vi "print.vi"(8 "error in (no error)":errorcluster, 10 "input":string, 11 "XMLPrettyPrinting in":refnum<class "XMLPrettyPrinting.lvclass">) -> (0 "error out":errorcluster, 2 "output":string, 3 "XMLPrettyPrinting out":refnum<class "XMLPrettyPrinting.lvclass">)   [LabVIEW 2011, in "Views.lvlib" / "ViewerTools.lvlib" / "XMLPrettyPrinting.lvclass"]
uses:
  XMLPrettyPrinting.lvclass
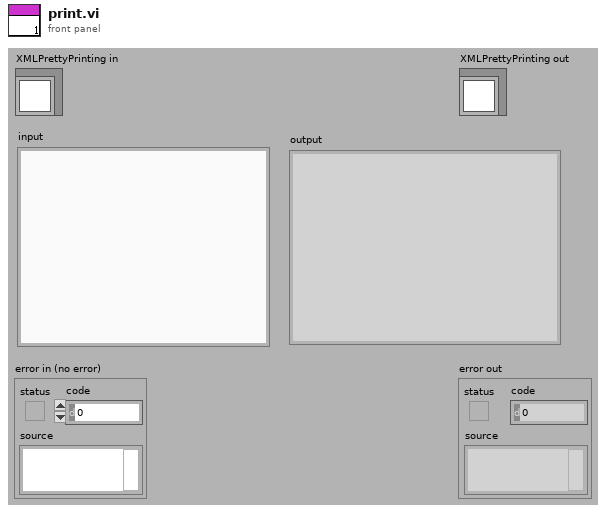
[diagram p1: front panel]
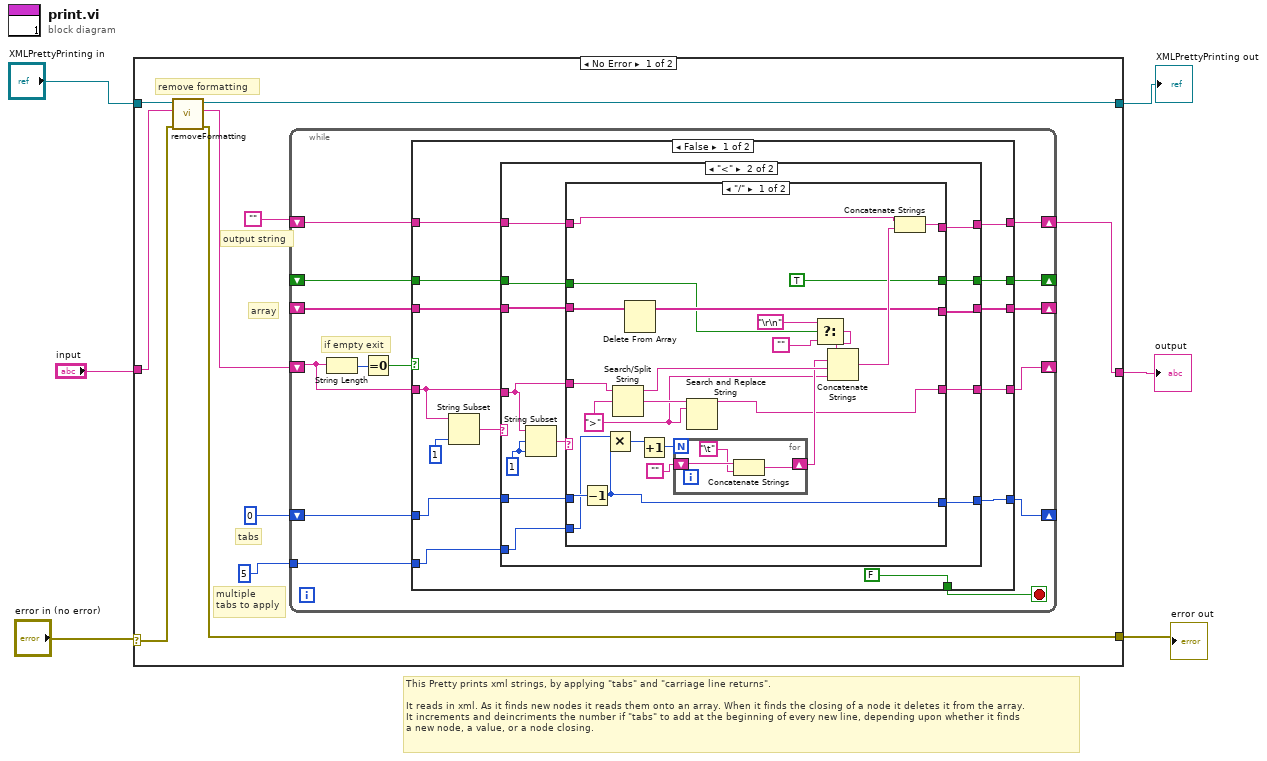
[diagram p0: block diagram]
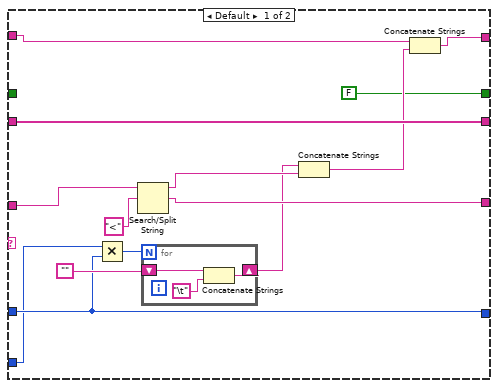
[diagram p2: hidden frame]
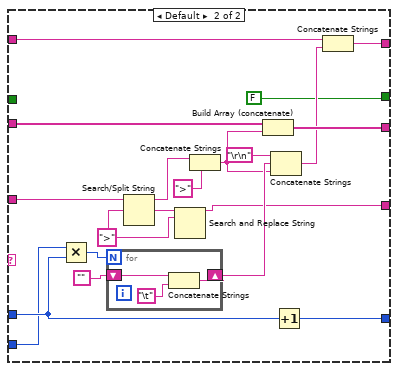
[diagram p3: hidden frame]
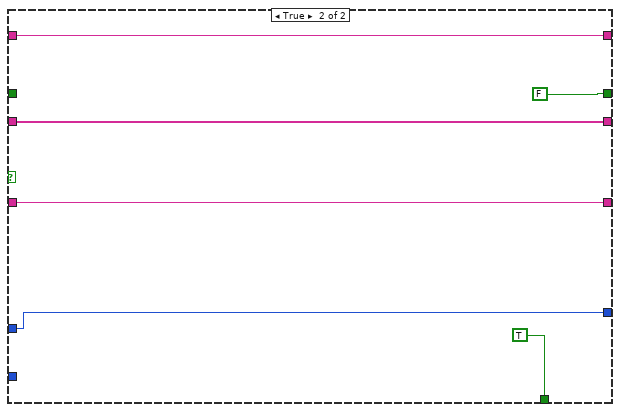
[diagram p4: hidden frame]
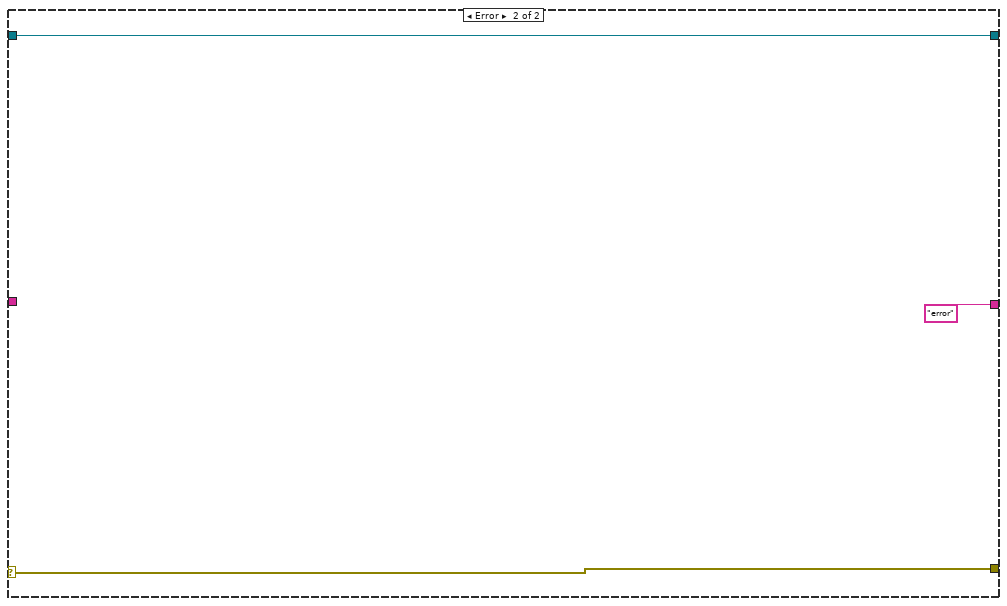
[diagram p5: hidden frame]
diagram:
  # "This Pretty prints xml strings, by applying \"tabs\" and \"carriage line returns\".\n\nIt reads in xml. As it finds new nodes it reads them onto an array. When it finds the closing of a node it deletes it from the array.\nIt increments and deincriments the number if \"tabs\" to add at the beginning of every new line, depending upon whether it finds\na new node, a value, or a node closing."
  n1 = case shown="No Error" "error in (no error)" {
    selector: "error in (no error)" -> [w10 w129]
    tunnel: [w9 w129] -> w5
    tunnel: "XMLPrettyPrinting in" -> [w12 w130]
    tunnel: [w7 w130] -> w3
    tunnel: "input" -> [w11 _]
    tunnel: [w14 "error"] -> w1
    frame No Error {
      # "remove formatting"
      # "output string"
      # "array"
      # "multiple\ntabs to apply"
      # "tabs"
      n2 = call-dynamic "removeFormatting.vi"("error in (no error)"=w10, "input"=w11, "XMLPrettyPrinting in"=w12) -> ("error out"=w9:errorcluster, "output"=w8:string, "XMLPrettyPrinting out"=w7:refnum<class "XMLPrettyPrinting.lvclass">)  [unwired: 6 in]
      n3 = while {
        shift-right: [w26] -> _
        shift-left: w8 -> [w28]
        shift-right: [w24] -> w14
        shift-left: "" -> [w25]
        shift-right: [w21] -> _
        shift-left: _ -> [w22]
        shift-right: [w20] -> _
        shift-left: 0 -> [w23]
        tunnel: 5 -> [w19]
        shift-right: [w18] -> _
        shift-left: _ -> [w17]
        stop <- w27 stop-if-true
        # "if empty exit"
        n4 = String Length(string=w28) -> (length=w30:i32)
        n5 = Equal To 0?(x=w30) -> (x = 0?=w29:bool)
        n6 = case shown="False" w29 {
          tunnel: w28 -> [w41 w127]
          tunnel: [FALSE TRUE] -> w27
          tunnel: [w34 w127] -> w26
          tunnel: w25 -> [w38 w126]
          tunnel: [w36 w126] -> w24
          tunnel: w23 -> [w37 w124]
          tunnel: w22 -> [w40 w125]
          tunnel: [w39 w125] -> w21
          tunnel: [w35 w124] -> w20
          tunnel: w19 -> [w33 _]
          tunnel: [w32 FALSE] -> w18
          tunnel: w17 -> [w31 _]
          frame False {
            n7 = String Subset(string=w41, length (rest)=1) -> (substring=w42:string)  [unwired: 1 in]
            n8 = case shown="\"<\"" w42 {
              tunnel: w41 -> [w56 w66]
              tunnel: w40 -> [w58 w74]
              tunnel: [w58 w73] -> w39
              tunnel: w38 -> [w48 w70]
              tunnel: w37 -> [w46 w72]
              tunnel: [w51 w69] -> w36
              tunnel: [w46 w71] -> w35
              tunnel: [w54 w68] -> w34
              tunnel: w33 -> [w45 w64]
              tunnel: [FALSE w63] -> w32
              tunnel: w31 -> [_ w62]
              frame Default {
                n9 = Multiply(x=w45, y=w46) -> (x*y=w47:i32)
                n10 = Search/Split String(string=w56, search string/char (-)="<") -> (substring before match=w53:string, match + rest of string=w54:string)  [unwired: 1 in, 1 out]
                n11 = for {
                  N: w47 -> [_]
                  shift-right: [w59] -> w52
                  shift-left: "" -> [w61]
                  n12 = Concatenate Strings(w61, "\t") -> (w59:string)
                }
                n13 = Concatenate Strings(w52, w53) -> (w50:string)
                n14 = Concatenate Strings(w48, w50) -> (w51:string)
              }
              frame "<" {
                w65 = 1
                n15 = String Subset(string=w66, offset (0)=w65, length (rest)=w65) -> (substring=w67:string)
                n16 = case shown="\"/\"" w67 {
                  tunnel: w66 -> [w91 w119]
                  tunnel: w74 -> [w89 w114]
                  tunnel: [w88 w113] -> w73
                  tunnel: w72 -> [w86 w105]
                  tunnel: [w78 w104] -> w71
                  tunnel: w70 -> [w79 w111]
                  tunnel: [w85 w110] -> w69
                  tunnel: [w87 w106] -> w68
                  tunnel: w64 -> [w76 w102]
                  tunnel: [TRUE FALSE] -> w63
                  tunnel: w62 -> [w82 _]
                  frame "/" {
                    w90 = ">"
                    n17 = Decrement(x=w86) -> (x-1=w78:i32)
                    n18 = Multiply(x=w76, y=w78) -> (x*y=w77:i32)
                    n19 = Search/Split String(string=w91, search string/char (-)=w90) -> (substring before match=w96:string, match + rest of string=w95:string)  [unwired: 1 in, 1 out]
                    n20 = Delete From Array(array=w89) -> (array with subset deleted=w88:string[])  [unwired: 2 in, 1 out]
                    n21 = Increment(x=w77) -> (x+1=w75:i32)
                    n22 = for {
                      N: w75 -> [_]
                      shift-right: [w97] -> w93
                      shift-left: "" -> [w99]
                      n23 = Concatenate Strings(w99, "\t") -> (w97:string)
                    }
                    n24 = Search and Replace String(input string=w95, search string=w90) -> (result string=w87:string)  [unwired: 6 in, 3 out]
                    n25 = Select(t="\r\n", s=w82, f="") -> (s? t:f=w81:string)
                    n26 = Concatenate Strings(w81, w93, w96, w90) -> (w92:string)
                    n27 = Concatenate Strings(w79, w92) -> (w85:string)
                  }
                  frame Default {
                    w118 = ">"
                    n28 = Multiply(x=w102, y=w105) -> (x*y=w103:i32)
                    n29 = for {
                      N: w103 -> [_]
                      shift-right: [w120] -> w109
                      shift-left: "" -> [w122]
                      n30 = Concatenate Strings(w122, "\t") -> (w120:string)
                    }
                    n31 = Search/Split String(string=w119, search string/char (-)=w118) -> (substring before match=w115:string, match + rest of string=w117:string)  [unwired: 1 in, 1 out]
                    n32 = Search and Replace String(input string=w117, search string=w118) -> (result string=w106:string)  [unwired: 6 in, 3 out]
                    n33 = Concatenate Strings(w115, ">") -> (w108:string)
                    n34 = Build Array (concatenate)(w114, w108) -> (w113:string[])
                    n35 = Concatenate Strings("\r\n", w109, w108) -> (w107:string)
                    n36 = Increment(x=w105) -> (x+1=w104:i32)
                    n37 = Concatenate Strings(w111, w107) -> (w110:string)
                  }
                }
              }
            }
          }
          frame True {
          }
        }
      }
    }
    frame Error {
    }
  }
  "error out" <- w5
  "XMLPrettyPrinting out" <- w3
  "output" <- w1
